vi "CS++RTCoreContent.vi"() -> (0 "CS++Classes & Messages":T1(array[cluster]))   [LabVIEW 2014]
doc: "This VI contains CS++Base Actors, Classes and Libs that can be used on RT."
uses:
  <vilib>/ActorFramework/Message/Message.lvclass
  CSPP_Core/Classes/CS++BaseClasses/Base/CS++Base.lvclass
  CSPP_Core/Classes/CS++BaseClasses/Factory/CS++Factory.lvclass
  CSPP_Core/Classes/CS++BaseClasses/Reference/CS++Reference.lvclass
  CSPP_Core/Classes/CS++BaseClasses/MessageLogger/CS++MessageLogger.lvclass
  CSPP_Core/Actors/CS++BaseActor/CS++BaseActor.lvclass
  CSPP_Core/Actors/CS++ControllerActor/CS++ControllerActor.lvclass
  CSPP_Core/Actors/CS++DeviceActor/CS++DeviceActor.lvclass
  CSPP_Core/Actors/CS++PVMonitor/CS++PVMonitor.lvclass
  CSPP_Core/Actors/CS++SVMonitor/CS++SVMonitor.lvclass
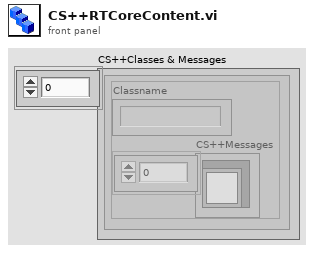
[diagram p1: front panel]
types:
  T1 = cluster{"Classname":string, "CS++Messages":refnum<class "Message.lvclass">[]}[]
  T2 = cluster{"class name":string, "CS++Messages":refnum<class "Message.lvclass">[]}
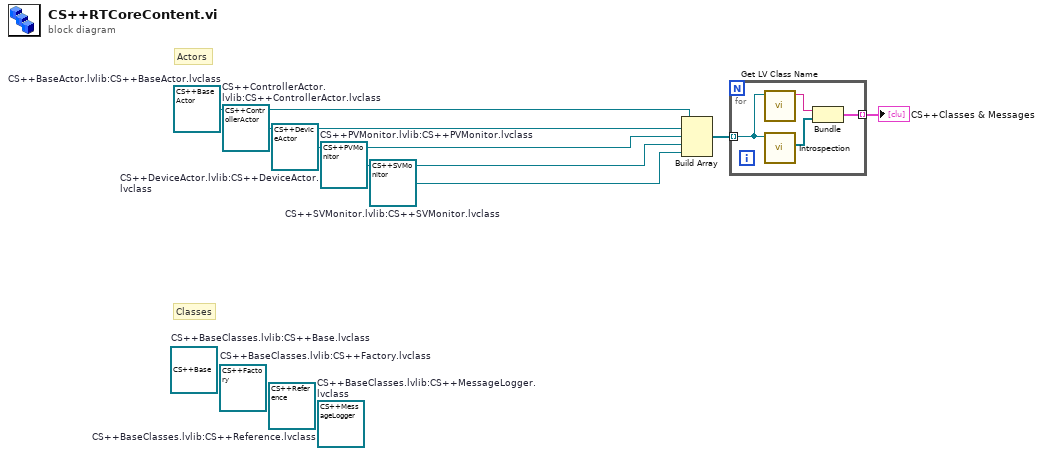
[diagram p0: block diagram]
diagram:
  w1 = refnum<class "CS++SVMonitor.lvclass"> refnum  # CS++SVMonitor.lvlib:CS++SVMonitor.lvclass
  w2 = refnum<class "CS++PVMonitor.lvclass"> refnum  # CS++PVMonitor.lvlib:CS++PVMonitor.lvclass
  w3 = refnum<class "CS++DeviceActor.lvclass"> refnum  # CS++DeviceActor.lvlib:CS++DeviceActor.lvclass
  w4 = refnum<class "CS++ControllerActor.lvclass"> refnum  # CS++ControllerActor.lvlib:CS++ControllerActor.lvclass
  w5 = refnum<class "CS++BaseActor.lvclass"> refnum  # CS++BaseActor.lvlib:CS++BaseActor.lvclass
  (unwired) refnum<class "CS++MessageLogger.lvclass"> refnum  # CS++BaseClasses.lvlib:CS++MessageLogger.lvclass
  (unwired) refnum<class "CS++Reference.lvclass"> refnum  # CS++BaseClasses.lvlib:CS++Reference.lvclass
  (unwired) refnum<class "CS++Factory.lvclass"> refnum  # CS++BaseClasses.lvlib:CS++Factory.lvclass
  (unwired) refnum<class "CS++Base.lvclass"> refnum  # CS++BaseClasses.lvlib:CS++Base.lvclass
  # "Actors"
  # "Classes"
  n1 = Build Array(w5, w4, w3, w2, w1) -> (w7:refnum<class "CS++BaseActor.lvclass">[])
  n2 = for {
    tunnel: w7 -> [w11] mode=indexing
    tunnel: [w8] -> w6 mode=indexing
    n3 = call <vilib>:"Get LV Class Name.vi"("object"=w11) -> ("class name"=w10:string)  [unwired: 9 in, 1 out]
    n4 = call "Introspection.vi"("CS++BaseActor in"=w11) -> ("CS++Messages"=w9:refnum<class "Message.lvclass">[])  [unwired: 8 in, 2 out]
    n5 = Bundle("class name"=w10, "CS++Messages"=w9) -> (w8:T2)  [unwired: 1 in]
  }
  "CS++Classes & Messages" <- w6
